vi "Trigger Continuous.vi"(6 "Settle (1mS)":u32=1, 8 "error in (no error)":errorcluster, 10 "Continuous Trigger (F: Off)":bool, 11 "VISA resource name":refnum<visa-resource-name>) -> (0 "error out":errorcluster, 3 "VISA resource name out":refnum<visa-resource-name>)   [LabVIEW 2018, in "TDK-Lambda Z.lvlib"]
doc: "Initiates transient generator trigger system.The function makes the trigger system change from idle state to waiting-for-trigger state. \n\nNote: This VI will wait for \"Settle\" milliseconds after setting the limit to allow the output to reach the new setting. If unwired, there will be no delay"
uses:
  TDK-Lambda Z.lvlib
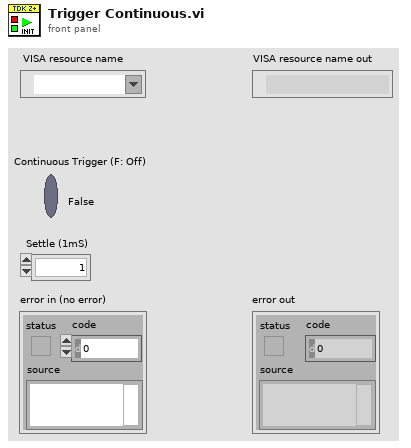
[diagram p1: front panel]
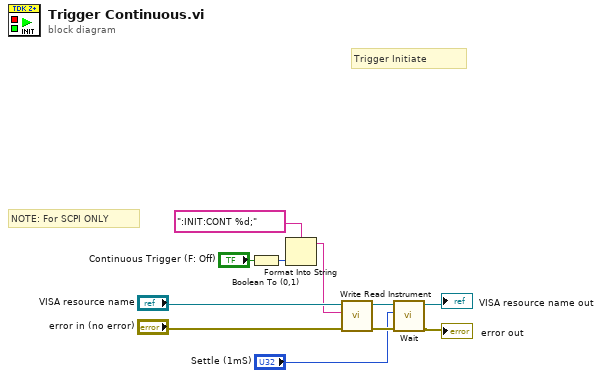
[diagram p0: block diagram]
diagram:
  # "NOTE: For SCPI ONLY"
  # "Trigger Initiate"
  n1 = Boolean To (0,1)(Boolean="Continuous Trigger (F: Off)") -> (0, 1=w2:i16)
  n2 = Format Into String(format string=":INIT:CONT %d;", w2) -> (resulting string=w1:string)  [unwired: 2 in, 1 out]
  n3 = call "Write Read Instrument.vi"("error in (no error)"="error in (no error)", "SCPI  Write Command/Query"=w1, "VISA resource name"="VISA resource name") -> ("error out"=w8:errorcluster, "VISA resource name out"=w9:refnum<visa-resource-name>)  [unwired: 6 in, 1 out]
  n4 = call "Wait.vi"("error in (no error)"=w8, "Wait (1mS)"="Settle (1mS)", "VISA resource name"=w9) -> ("error out"=→"error out":errorcluster, "VISA resource name out"=→"VISA resource name out":refnum<visa-resource-name>)  [unwired: 7 in]
